vi "Deembedding RFmx.vi"(7 "Selector String":string, 8 "error in":errorcluster, 11 "RFmx Settings":T1={"RFmx Name"="5842_0", "RFmx Port"="", "Attenuation"={"Mode"=enum."Constant Attenuation", "Constant Attenuation"={"RFmx External Attenuation (dB)"=1.2}, "s2p File"={"RFmx S-Parameters Orientation"=24000, "RFmx Attenuation s2p Path Name"="", "RFmx Attenuation s2p File"=path ""}}} {"Attenuation"."s2p File"."RFmx S-Parameters Orientation" items=["Port1 Towards DUT"=24000, "Port2 Towards DUT"=24001]; "Attenuation"."Constant Attenuation"."RFmx External Attenuation (dB)" format="%.2f"}) -> (0 "error out":errorcluster, 3 "Refnum out":refnum<k21>)   [LabVIEW 2023]
uses:
  RFmx Config.ctl
  <vilib>/RFmx/RFInstr/mx/RFmxInstr.llb/RFmxInstr Configure External Attenuation Interpolation (Nearest).vi
panel:
  out "Created New?":bool
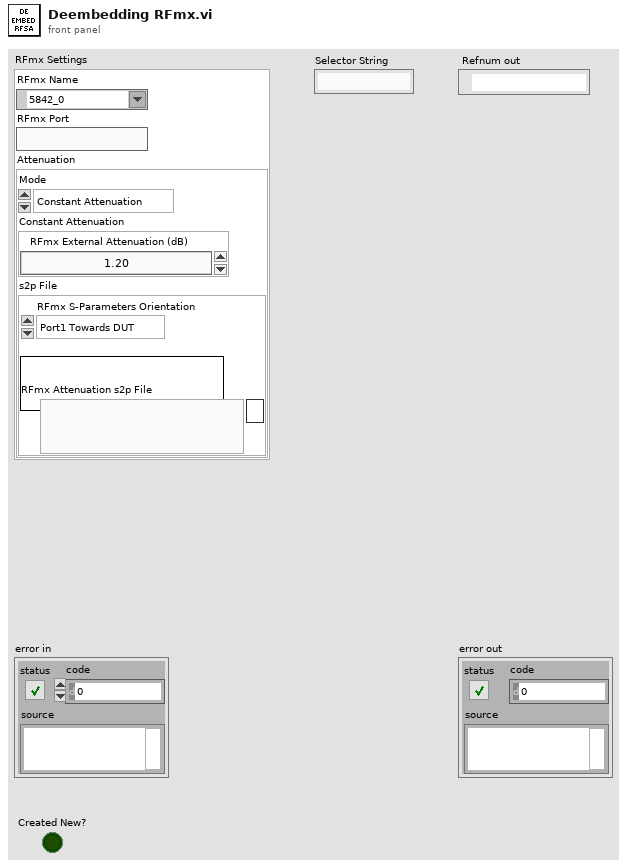
[diagram p1: front panel]
types:
  T1 = typedef "RFmx Config.ctl" = cluster{"RFmx Name":refnum<k15>, "RFmx Port":string, "Attenuation":cluster{"Mode":enum32{"<None>", "Constant Attenuation", "s2p File"}, "Constant Attenuation":cluster{"RFmx External Attenuation (dB)":dbl}, "s2p File":cluster{"RFmx S-Parameters Orientation":i32, "RFmx Attenuation s2p Path Name":string, "RFmx Attenuation s2p File":path}}}
  T2 = enum32{"<None>", "Constant Attenuation", "s2p File"}
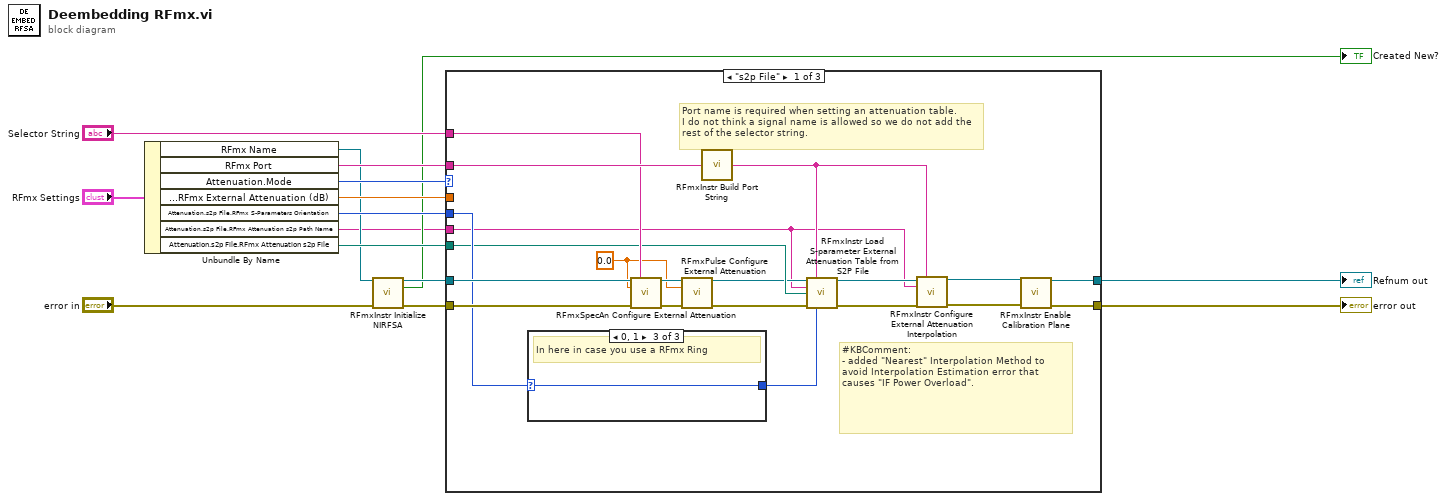
[diagram p0: block diagram]
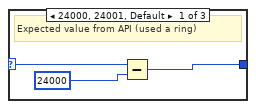
[diagram p2: hidden frame]
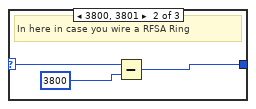
[diagram p3: hidden frame]
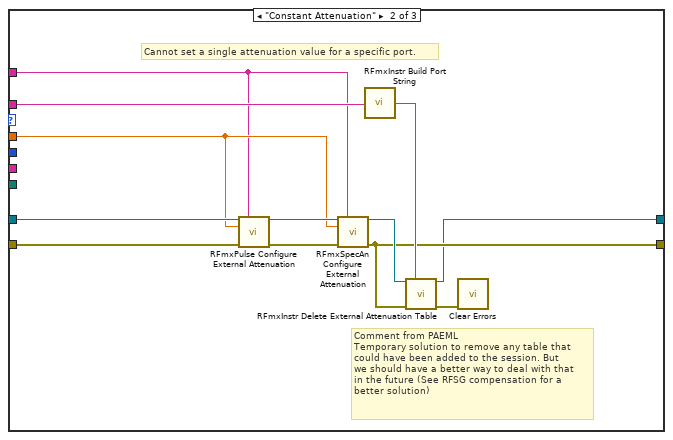
[diagram p4: hidden frame]
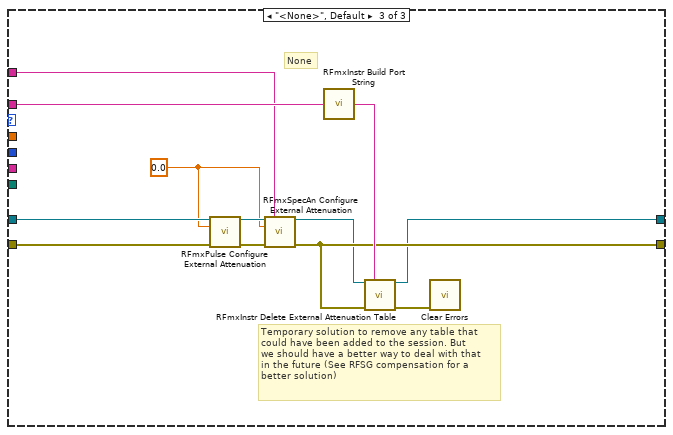
[diagram p5: hidden frame]
diagram:
  n1 = Unbundle By Name("RFmx Settings") -> ("RFmx Name"=w2:refnum<k15>, "RFmx Port"=w12:string, "Attenuation.Mode"=w10:T2, "Attenuation.Constant Attenuation.RFmx External Attenuation (dB)"=w11:dbl, "Attenuation.s2p File.RFmx S-Parameters Orientation"=w9:i32, "Attenuation.s2p File.RFmx Attenuation s2p Path Name"=w1:string, "Attenuation.s2p File.RFmx Attenuation s2p File"=w8:path)
  n2 = call <vilib>:"RFmxInstr Initialize NIRFSA.vi"("Resource Name"=w2, "error in (no error)"="error in") -> ("Instrument Handle Out"=w13:refnum<k21>, "Created New?"=→"Created New?":bool, "error out"=w6:errorcluster)  [unwired: 11 in]
  n3 = case shown="\"s2p File\"" w10 {
    tunnel: w13 -> [w33 w47 w57]
    tunnel: w6 -> [w34 w48 w56]
    tunnel: [w31 w49 w60] -> w4
    tunnel: [w30 w50 w63] -> w3
    tunnel: w9 -> [w29 _ _]
    tunnel: w11 -> [_ w44 _]
    tunnel: "Selector String" -> [w32 w43 w62]
    tunnel: w12 -> [w35 w52 w66]
    tunnel: w8 -> [w27 _ _]
    tunnel: w1 -> [w16 _ _]
    frame "s2p File" {
      w22 = 0.0 ("External Attenuation (dB)")
      # "#KBComment:\n- added \"Nearest\" Interpolation Method to avoid Interpolation Estimation error that causes \"IF Power Overload\"."
      # "Port name is required when setting an attenuation table.\nI do not think a signal name is allowed so we do not add the rest of the selector string."
      n4 = case shown="0, 1" w29 {
        selector: w29 -> [w38 w41 w42]
        tunnel: [w36 w39 w42] -> w28
        frame 24000, 24001, Default {
          # "Expected value from API (used a ring)"
          n5 = Subtract(x=w38, y=24000) -> (x-y=w36:i32)
        }
        frame 3800, 3801 {
          # "In here in case you wire a RFSA Ring"
          n6 = Subtract(x=w41, y=3800) -> (x-y=w39:i32)
        }
        frame 0, 1 {
          # "In here in case you use a RFmx Ring"
        }
      }
      n7 = call <vilib>:"RFmxSpecAn Configure External Attenuation.vi"("Instrument Handle In"=w33, "Selector String"=w32, "External Attenuation (dB)"=w22, "error in (no error)"=w34) -> ("Instrument Handle Out"=w26:refnum<k21>, "error out"=w25:errorcluster)  [unwired: 10 in]
      n8 = call <vilib>:"RFmxPulse Configure External Attenuation.vi"("Instrument Handle In"=w26, "External Attenuation (dB)"=w22, "error in (no error)"=w25) -> ("Instrument Handle Out"=w24:refnum<k21>, "error out"=w23:errorcluster)  [unwired: 11 in]
      n9 = call <vilib>:"RFmxInstr Build Port String.vi"("Port Name"=w35) -> ("Selector String Out"=w17:string)  [unwired: 14 in]
      n10 = call <vilib>:"RFmxInstr Load S-parameter External Attenuation Table from S2P File.vi"("Instrument Handle In"=w24, "Selector String"=w17, "Table Name"=w16, "S2P File Path"=w27, "error in (no error)"=w23, "S-parameter Orientation"=w28) -> ("Instrument Handle Out"=w21:refnum<k21>, "error out"=w20:errorcluster)  [unwired: 8 in]
      n11 = call-poly <vilib>:"RFmxInstr Configure External Attenuation Interpolation.vi"("Instrument Handle In"=w21, "Selector String"=w17, "Table Name"=w16, "error in (no error)"=w20) -> ("Instrument Handle Out"=w19:refnum<k21>, "error out"=w18:errorcluster)  [unwired: 10 in]
      n12 = call <vilib>:"RFmxInstr Enable Calibration Plane.vi"("Instrument Handle In"=w19, "error in (no error)"=w18) -> ("Instrument Handle Out"=w31:refnum<k21>, "error out"=w30:errorcluster)  [unwired: 12 in]
    }
    frame "Constant Attenuation" {
      # "Comment from PAEML\nTemporary solution to remove any table that \ncould have been added to the session. But\nwe should have a better way to deal with that\nin the future (See RFSG compensation for a \nbetter solution)"
      # "Cannot set a single attenuation value for a specific port."
      n13 = call <vilib>:"RFmxPulse Configure External Attenuation.vi"("Instrument Handle In"=w47, "Selector String"=w43, "External Attenuation (dB)"=w44, "error in (no error)"=w48) -> ("Instrument Handle Out"=w46:refnum<k21>, "error out"=w45:errorcluster)  [unwired: 10 in]
      n14 = call <vilib>:"RFmxSpecAn Configure External Attenuation.vi"("Instrument Handle In"=w46, "Selector String"=w43, "External Attenuation (dB)"=w44, "error in (no error)"=w45) -> ("Instrument Handle Out"=w51:refnum<k21>, "error out"=w50:errorcluster)  [unwired: 10 in]
      n15 = call <vilib>:"RFmxInstr Build Port String.vi"("Port Name"=w52) -> ("Selector String Out"=w54:string)  [unwired: 14 in]
      n16 = call <vilib>:"RFmxInstr Delete External Attenuation Table.vi"("Instrument Handle In"=w51, "Selector String"=w54, "error in (no error)"=w50) -> ("Instrument Handle Out"=w49:refnum<k21>, "error out"=w53:errorcluster)  [unwired: 11 in]
      n17 = call <vilib>:"Clear Errors.vi"("error in (no error)"=w53) -> ()  [unwired: 5 in, 2 out]
    }
    frame "<None>", Default {
      w55 = 0.0 ("External Attenuation (dB)")
      # "None"
      # "Temporary solution to remove any table that \ncould have been added to the session. But\nwe should have a better way to deal with that\nin the future (See RFSG compensation for a \nbetter solution)"
      n18 = call <vilib>:"RFmxPulse Configure External Attenuation.vi"("Instrument Handle In"=w57, "External Attenuation (dB)"=w55, "error in (no error)"=w56) -> ("Instrument Handle Out"=w59:refnum<k21>, "error out"=w58:errorcluster)  [unwired: 11 in]
      n19 = call <vilib>:"RFmxSpecAn Configure External Attenuation.vi"("Instrument Handle In"=w59, "Selector String"=w62, "External Attenuation (dB)"=w55, "error in (no error)"=w58) -> ("Instrument Handle Out"=w61:refnum<k21>, "error out"=w63:errorcluster)  [unwired: 10 in]
      n20 = call <vilib>:"RFmxInstr Build Port String.vi"("Port Name"=w66) -> ("Selector String Out"=w65:string)  [unwired: 14 in]
      n21 = call <vilib>:"RFmxInstr Delete External Attenuation Table.vi"("Instrument Handle In"=w61, "Selector String"=w65, "error in (no error)"=w63) -> ("Instrument Handle Out"=w60:refnum<k21>, "error out"=w64:errorcluster)  [unwired: 11 in]
      n22 = call <vilib>:"Clear Errors.vi"("error in (no error)"=w64) -> ()  [unwired: 5 in, 2 out]
    }
  }
  "error out" <- w3
  "Refnum out" <- w4
